vi "ifr2025 Control.vi"(8 "error in (no error)":errorcluster {"code" format="%.0x"}, 9 "Pulse (Off)":bool, 10 "Global Mod (Off)":bool, 11 "instrument handle":refnum<visa-resource-name>) -> (0 "error out":errorcluster {"code" format="%.0x"}, 3 "instrument handle out":refnum<visa-resource-name>)   [LabVIEW 2009]
doc: "Controls the global modes of modulation and pulse."
uses:
  Ifr2025_32.dll
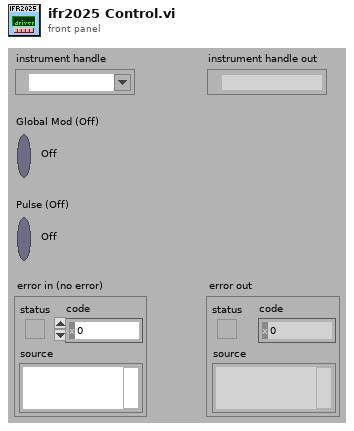
[diagram p1: front panel]
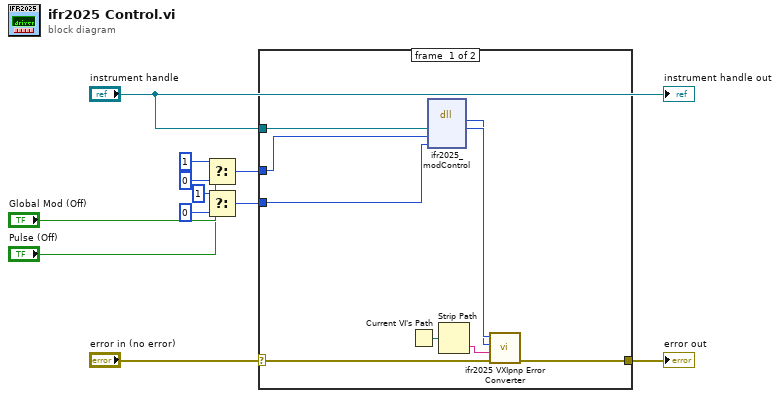
[diagram p0: block diagram]
diagram:
  n1 = Select(t=u16 1, s="Global Mod (Off)", f=u16 0) -> (s? t:f=w5:u16)
  n2 = Select(t=u16 1, s="Pulse (Off)", f=u16 0) -> (s? t:f=w1:u16)
  n3 = case shown="No Error" "error in (no error)" {
    selector: "error in (no error)" -> [w15 w21]
    tunnel: [w14 w21] -> w11
    tunnel: "instrument handle" -> [w19 _]
    tunnel: w5 -> [w13 _]
    tunnel: w1 -> [w12 _]
    frame #0 {
      n4 = Current VI's Path() -> (path=w20:path)
      n5 = dll-call lib="P:/inst/Marconi 2024 Signal Generator/source/labview/ifr2025/ifr2025/ifr2025_*.*" fn="ifr2025_modControl"("vi"=w19, "Global Mod"=w13, "Pulse"=w12) -> (w17:i32, "vi"=w18:u32)  [unwired: 5 in, 2 out]
      n6 = Strip Path(path=w20) -> (name=w16:string)  [unwired: 1 out]
      n7 = call "ifr2025 VXIpnp Error Converter.vi"("error in (no error)"=w15, "name of VI (\"\")"=w16, "CVI error code (0)"=w17, "instrument handle"=w18) -> ("error out"=w14:errorcluster)  [unwired: 7 out]
    }
    frame #1 {
    }
  }
  "error out" <- w11
  "instrument handle out" <- "instrument handle"
